vi "Event 2 Mouse Down.vi"   [LabVIEW 2014]
uses:
  Controls/GMap Mouse States.ctl
  FGVs/GMap Mouse State/Methods/SET Mouse State.vi
types:
  T1 = typedef "GMap Mouse States.ctl" = enum16{"Mouse Down", "Mouse Up"}
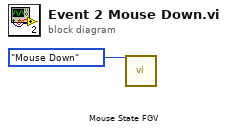
[diagram p0: block diagram]
diagram:
  n1 = call-poly "Mouse State FGV.vi"("Mouse State In"=GMap_Mouse_States."Mouse Down") -> ()  [unwired: 10 in, 1 out]
